vi "Convert string to bitmap.vi"(0 "data":string, 11 "error in (no error)":errorcluster) -> (4 "image data":T2, 15 "error out":errorcluster)   [LabVIEW 2017]
doc: "Reads a Windows bitmap file and creates the data necessary to display the file in a picture control."
uses:
  <vilib>/picture/picture.llb/imagedata.ctl
panel:
  out "BMP data":u8[](array[numeric])
  out "color table":u32[](array[colorbox])
  out "bitmap info":T1
  out "file type wrong":bool
  out "bitmap depth is wrong":bool
  out "bitmap is compressed":bool
  out "bitmap header wrong size":bool
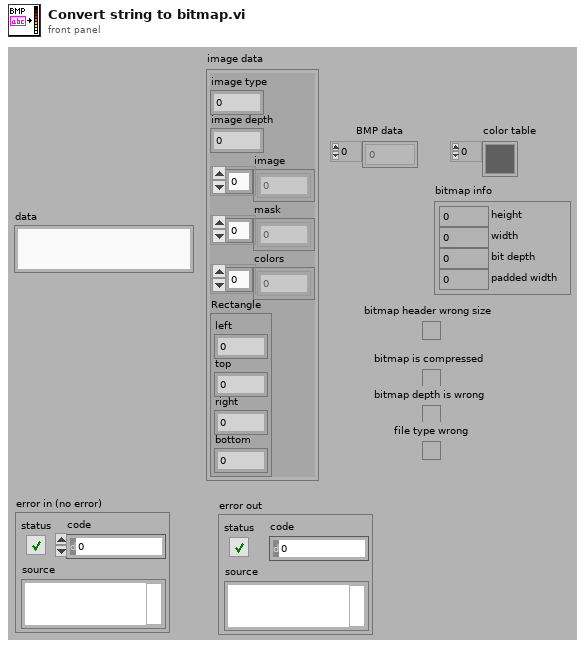
[diagram p1: front panel]
types:
  T1 = cluster{"height":u32, "width":u32, "bit depth":u16, "padded width":u32}
  T2 = typedef "imagedata.ctl" = cluster{"image type":i32, "image depth":i32, "image":u8[], "mask":u8[], "colors":u32[], "Rectangle":cluster{"left":i16, "top":i16, "right":i16, "bottom":i16}}
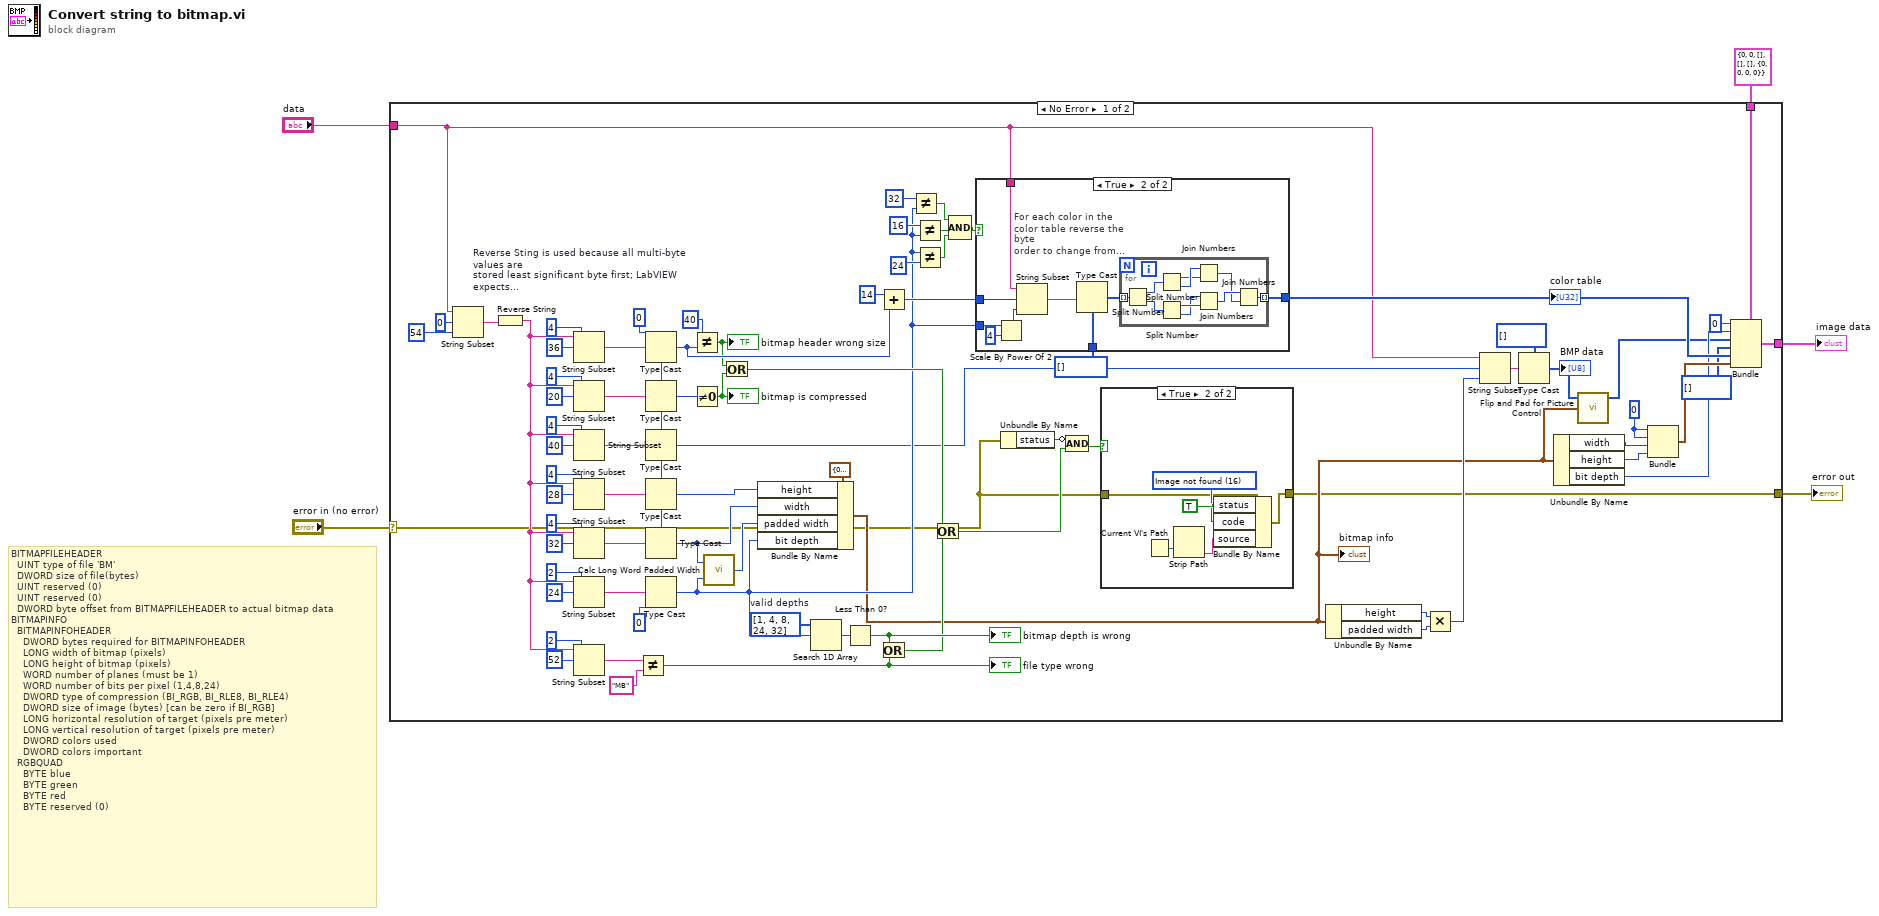
[diagram p0: block diagram]
diagram:
  # "BITMAPFILEHEADER\n  UINT\ttype of file 'BM'\n  DWORD\tsize of file(bytes)\n  UINT\treserved (0)\n  UINT\treserved (0)\n  DWORD\tbyte offset from BITMAPFILEHEADER to actual bitmap data\nBITMAPINFO\n  BITMAPINFOHEADER\n    DWORD\tbytes required for BITMAPINFOHEADER\n    LONG\twidth of bitmap (pixels)\n    LONG\theight of bitmap (pixels)\n    WORD\tnumber of planes (must be 1)\n    WORD\tnumber of bits per pixel (1,4,8,24)\n    DWORD\ttype of compression (BI_RGB, BI_RLE8, BI_RLE4)\n    DWORD\tsize of image (bytes) [can be zero if BI_RGB]\n    LONG\thorizontal resolution of target (pixels pre meter)\n    LONG\tvertical resolution of target (pixels pre meter)\n    DWORD\tcolors used\n    DWORD\tcolors important\n  RGBQUAD\n    BYTE\tblue\n    BYTE\tgreen\n    BYTE\tred\n    BYTE\treserved (0)"
  n1 = case shown="No Error" "error in (no error)" {
    selector: "error in (no error)" -> [w6 w113]
    tunnel: T2 {"image type"=0, "image depth"=0, "image"=[], "mask"=[], "colors"=[], "Rectangle"={"left"=0, "top"=0, "right"=0, "bottom"=0}} ("image data 2") -> [w84 w112]
    tunnel: [w83 w112] -> w4
    tunnel: "data" -> [w16 _]
    tunnel: [w7 w113] -> w2
    frame No Error {
      w15 = i16 0
      w64 = u32[] [1, 4, 8, 24, 32]  # valid depths
      w50 = u32 0 ("uint32")
      n2 = String Subset(string=w16, offset (0)=0, length (rest)=54) -> (substring=w23:string)
      n3 = Reverse String "Reverse Sting is used because all multi-byte values are\nstored least significant byte first; LabVIEW expects \nmost significant byte first."(1:w23) -> (0:w48:string)
      n4 = String Subset(string=w48, offset (0)=36, length (rest)=4) -> (substring=w47:string)
      n5 = String Subset(string=w48, offset (0)=20, length (rest)=4) -> (substring=w46:string)
      n6 = String Subset(string=w48, offset (0)=40, length (rest)=4) -> (substring=w45:string)
      n7 = String Subset(string=w48, offset (0)=28, length (rest)=4) -> (substring=w44:string)
      n8 = String Subset(string=w48, offset (0)=32, length (rest)=4) -> (substring=w43:string)
      n9 = String Subset(string=w48, offset (0)=24, length (rest)=2) -> (substring=w42:string)
      n10 = String Subset(string=w48, offset (0)=52, length (rest)=2) -> (substring=w52:string)
      n11 = Not Equal?(x=w52, y="MB") -> (x != y?=w59:bool)
      "file type wrong" <- w59
      n12 = Type Cast(type=w50, x=w47) -> (*(type *) &x=w71:u32)
      n13 = Type Cast(type=w50, x=w46) -> (*(type *) &x=w68:u32)
      n14 = Type Cast(type=w50, x=w45) -> (*(type *) &x=w22:u32)
      n15 = Type Cast(type=w50, x=w44) -> (*(type *) &x=w55:u32)
      n16 = Type Cast(type=w50, x=w43) -> (*(type *) &x=w54:u32)
      n17 = Type Cast(type=u16 0 ("uint16"), x=w42) -> (*(type *) &x=w30:u16)
      n18 = Not Equal?(x=40, y=w71) -> (x != y?=w67:bool)
      "bitmap header wrong size" <- w67
      n19 = Not Equal To 0?(x=w68) -> (x != 0?=w66:bool)
      "bitmap is compressed" <- w66
      n20 = call <vilib>:"Calc Long Word Padded Width.vi"("bit depth"=w30, "width"=w54) -> ("padded width"=w53:i32)
      n21 = Or(x=w67, y=w66) -> (x .or. y?=w65:bool)
      n22 = Bundle By Name(cluster=T1 {"height"=0, "width"=0, "bit depth"=0, "padded width"=0} ("used for datatype only"), "height"=w55, "width"=w54, "padded width"=w53, "bit depth"=w30) -> (w17:T1)
      "bitmap info" <- w17
      n23 = Search 1D Array(1D array=w64, element=w30) -> (index of element=w63:i32)  [unwired: 1 in]
      n24 = Less Than 0?(x=w63) -> (x < 0?=w58:bool)
      "bitmap depth is wrong" <- w58
      n25 = Add(x=14, y=w71) -> (x+y=w72:u32)
      n26 = Or(x=w58, y=w59) -> (x .or. y?=w57:bool)
      n27 = Not Equal?(x=u16 32, y=w30) -> (x != y?=w29:bool)
      n28 = Not Equal?(x=u16 16, y=w30) -> (x != y?=w35:bool)
      n29 = Not Equal?(x=w30, y=24) -> (x != y?=w34:bool)
      n30 = Or(x=w65, y=w57) -> (x .or. y?=w40:bool)
      n31 = Compound Arithmetic op=AND(w29, w35, w34) -> (w33:bool)
      n32 = case shown="True" w33 {
        tunnel: [w85 w93] -> w18
        tunnel: w72 -> [_ w87]
        tunnel: u32[] [] ("color table") -> [w85 w92]
        tunnel: w30 -> [_ w91]
        tunnel: w16 -> [_ w88]
        frame False {
        }
        frame True {
          n33 = Scale By Power Of 2(n=w91, x=4) -> (x*2^n=w86:i32)
          n34 = String Subset(string=w88, offset (0)=w87, length (rest)=w86) -> (substring=w89:string)
          n35 = Type Cast(type=w92, x=w89) -> (*(type *) &x=w90:u32[])
          n36 = for "For each color in the color table reverse the byte\norder to change from  least significant byte first\nto most significant byte first." {
            tunnel: [w104] -> w93 mode=indexing
            tunnel: w90 -> [w95] mode=indexing
            n37 = Split Number(x=w95) -> (hi(x)=w102:u16, lo(x)=w103:u16)
            n38 = Split Number(x=w102) -> (hi(x)=w100:u8, lo(x)=w101:u8)
            n39 = Split Number(x=w103) -> (hi(x)=w99:u8, lo(x)=w98:u8)
            n40 = Join Numbers(hi=w101, lo=w100) -> ((hi.lo)=w96:u16)
            n41 = Join Numbers(hi=w98, lo=w99) -> ((hi.lo)=w97:u16)
            n42 = Join Numbers(hi=w97, lo=w96) -> ((hi.lo)=w104:u32)
          }
        }
      }
      "color table" <- w18
      n43 = Unbundle By Name(w6) -> ("status"=w39:bool)
      n44 = Compound Arithmetic op=AND(invert w39, w40) -> (w38:bool)
      n45 = case shown="True" w38 {
        tunnel: [w105 w107] -> w7
        tunnel: w6 -> [w105 w106]
        frame False {
        }
        frame True {
          w110 = u16 16 items=["No error", "Argument error", "Memory is full", "Out of zone", "End of file", "File already open", "Generic file I/O error", "File not found", "File permission error", "Disk is full", "Duplicate path", "Too many files open", "System feature not enabled", "Resource file not found", "Cannot add resource", "Resource not found", "Image not found", "Image memory error", "Pen does not exist", "Config type invalid", "Config token not found", "Config parse error", "Config memory error", "Bad external code format", "Bad external code offset", "External code not present", "Null window", "Destroy window error", "Null menu", "Print aborted", "Bad print record", "Print driver error", "Windows error during printing", "Memory error during printing", "Print dialog error", "Generic print error", "Invalid device refnum", "Device not found", "Device parameter error", "Device unit error", "Cannot open device", "Device call aborted", "Generic error", "Cancelled by user", "Object ID too low", "Object ID too high", "Object not in heap", "Unknown heap", "Unknown object (invalid DefProc)", "Unknown object (DefProc not in table)", "Message out of range", "Invalid (null) method", "Unknown message", "Manager call not supported", "Bad address", "Network operation in progress", "Network operation timed out", "Connection is busy", "Network attribute not supported", "Network error", "Address in use", "System out of memory", "Connection aborted", "Connection refused", "Not connected", "Already connected", "Connection closed", "Initialization error (interapplication manager)", "Bad occurrence", "Wait on unbound occurrence handler", "Occurrence queue overflow", "Datalog type conflict", "Unused", "Unrecognized type (interapplication manager)", "Memory corrupt", "Failed to make temporary DLL", "Old CIN version", "Drag socket not found", "Failed to load drop-object", "Failed to register OLE object", "Failed to release OLE object", "Format specifier type mismatch", "Unknown format specifier", "Too few format specifiers", "Too many format specifiers", "Scan failed", "Newer CIN version", "OLE Convert", "Runtime menu error", "Password tampered", "Unknown error code"]
          n46 = Current VI's Path() -> (path=w108:path)
          n47 = Strip Path(path=w108) -> (name=w109:string)  [unwired: 1 out]
          n48 = Bundle By Name(cluster=w106, "status"=TRUE, "code"=w110, "source"=w109) -> (w107:errorcluster)
        }
      }
      n49 = Unbundle By Name(w17) -> ("height"=w24:u32, "padded width"=w26:u32)
      n50 = Multiply(x=w24, y=w26) -> (x*y=w21:u32)
      n51 = String Subset(string=w16, offset (0)=w22, length (rest)=w21) -> (substring=w20:string)
      n52 = Type Cast(type=u8[] [] ("array of bytes"), x=w20) -> (*(type *) &x=w19:u8[])
      "BMP data" <- w19
      n53 = Unbundle By Name(w17) -> ("width"=w14:u32, "height"=w13:u32, "bit depth"=w11:u16)
      n54 = call <vilib>:"Flip and Pad for Picture Control.vi"("bitmap info"=w17, "BMP bitmap"=w19) -> ("picture bitmap"=w8:u8[])  [unwired: 3 in]
      n55 = Bundle(w15, w15, "width"=w14, "height"=w13) -> (w12:cluster{i16, i16, "width":u32, "height":u32})  [unwired: 1 in]
      n56 = Bundle(cluster=w84, "image type"=0, "image depth"=w11, "image"=w8, "mask"=u8[] [] ("image"), "colors"=w18, "Rectangle"=w12) -> (w83:T2)
    }
    frame Error {
    }
  }
  "image data" <- w4
  "error out" <- w2
